vi "Write Teller Metadata.vi"(7 "Msg in":refnum<class "Msg.lvclass">, 10 "Teller Metadata":refnum<class "Teller Metadata.lvclass">) -> (5 "Msg out":refnum<class "Msg.lvclass">)   [LabVIEW 2020, in "jettl.lvlib"]
uses:
  jettl.lvlib
  Msg/Msg.lvclass
  Teller Metadata/Teller Metadata.lvclass
  Msg Input/Msg Input.lvclass
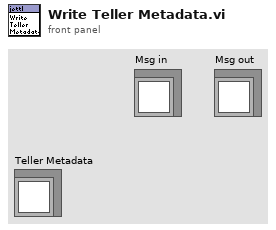
[diagram p1: front panel]
types:
  T1 = typedef "jettl.lvlib/Teller.ctl" = cluster{"Priority":bool, "Time":timestamp, "UID":i32, "Alias":string, "Valid Relation":bool, "Relation":T2, "Called From Msg Library":bool, "Teller Metadata":refnum<class "Teller Metadata.lvclass">}
  T2 = typedef "jettl.lvlib/Relation.ctl" = enum16{"Self", "Parent", "Child"}
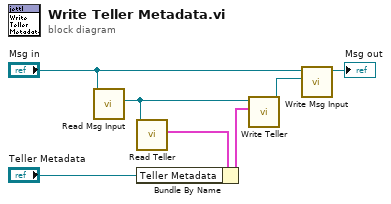
[diagram p0: block diagram]
diagram:
  n1 = call-dynamic "Read Msg Input.vi"("Msg in"="Msg in") -> ("Msg Input"=w4:refnum<class "Msg Input.lvclass">)  [unwired: 10 in]
  n2 = call-dynamic "Read Teller.vi"("Msg Input in"=w4) -> ("Teller"=w3:T1)  [unwired: 10 in]
  n3 = Bundle By Name(cluster=w3, "Teller Metadata"="Teller Metadata") -> (w2:T1)
  n4 = call-dynamic "Write Teller.vi"("Teller"=w2, "Msg Input in"=w4) -> ("Msg Input out"=w5:refnum<class "Msg Input.lvclass">)  [unwired: 9 in]
  n5 = call-dynamic "Write Msg Input.vi"("Msg Input"=w5, "Msg in"="Msg in") -> ("Msg out"=→"Msg out":refnum<class "Msg.lvclass">)  [unwired: 9 in]
